vi "Commit Calibration Data.vi"(0 "CART TCP Connection In":refnum<k5>, 11 "error in (no error)":errorcluster) -> (4 "CART TCP Connection Out":refnum<k5>, 8 "TCP Messages":string[](array[string]), 15 "error out":errorcluster)   [LabVIEW 2011]
uses:
  CART/Controls/Parameter.ctl
  SubVIs/NART Constants.vi
  ART2 Test Panel.lvlib
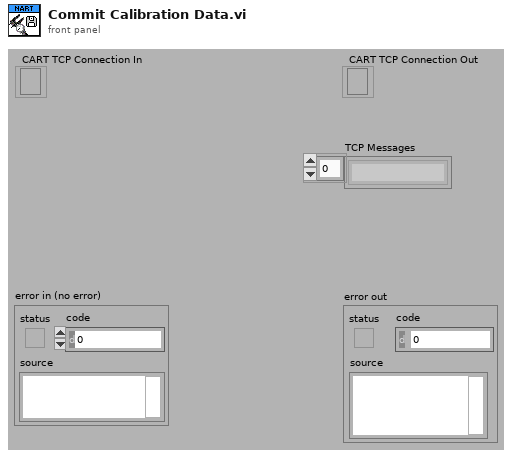
[diagram p1: front panel]
types:
  T1 = typedef "ART2 Test Panel.lvlib/Parameter.ctl" = cluster{"Name":string, "Type":enum16{"decimal", "string", "float", "hex"}}
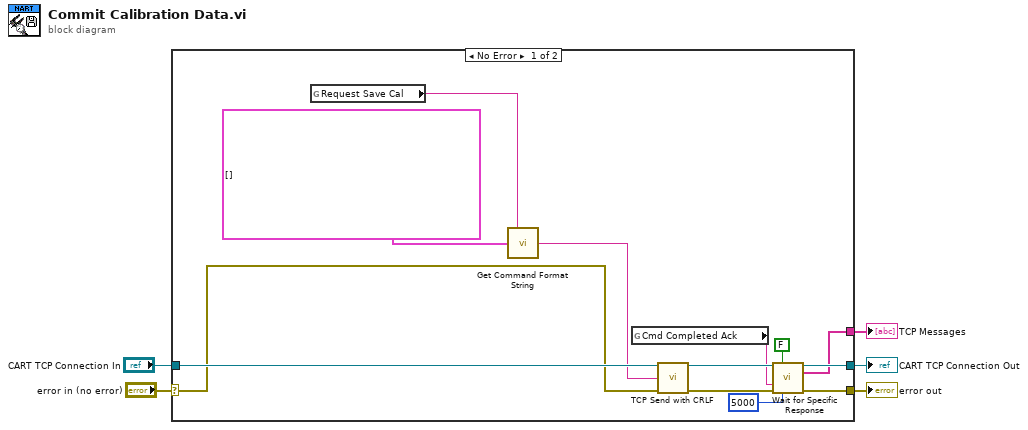
[diagram p0: block diagram]
diagram:
  n1 = case shown="No Error" "error in (no error)" {
    selector: "error in (no error)" -> [w15 w20]
    tunnel: [w12 w20] -> w4
    tunnel: "CART TCP Connection In" -> [w18 w19]
    tunnel: [w13 w19] -> w2
    tunnel: [w9 _] -> w1
    frame No Error {
      n2 = global read "NART Constants.vi" "Request Save Cal"() -> (w7:string)
      n3 = call "Get Command Format String.vi"("Command"=w7, "Parameters"=T1[] []) -> ("Command Format String"=w16:string)  [unwired: 13 in]
      n4 = global read "NART Constants.vi" "Cmd Completed Ack"() -> (w6:string)
      n5 = call "TCP Send with CRLF.vi"("CART TCP Connection"=w18, "data in"=w16, "error IO"=w15) -> ("CART TCP Connection Out"=w14:refnum<k5>, "error out"=w11:errorcluster)  [unwired: 11 in]
      n6 = call "Wait for Specific Response.vi"("TCP Connection In"=w14, "Next response (t)"=FALSE, "Expected Message Start (\"\":any)"=w6, "error in"=w11, "Timeout (250 ms)"=5000) -> ("TCP Connection Out"=w13:refnum<k5>, "TCP Messages"=w9:string[], "error out"=w12:errorcluster)  [unwired: 7 in, 1 out]
    }
    frame Error {
    }
  }
  "error out" <- w4
  "CART TCP Connection Out" <- w2
  "TCP Messages" <- w1
